vi "Format Geometric Patterns Results (SubVI).vi"(8 "error in":errorcluster, 11 "Matches":T1[](array[typedef]) {"Correlation Score" format="%.2f"; "Target Template Curve Score" format="%.2f"; "Template Target Curve Score" format="%.2f"; "Bounding Box"."y" format="%.2f"; "Bounding Box"."x" format="%.2f"; "Position"."y" format="%.2f"; "Position"."x" format="%.2f"; "Score" format="%.2f"; "Scale" format="%.2f"; "Angle" format="%.2f"; "Occlusion %" format="%.2f"}) -> (0 "error out":errorcluster, 3 "Text Results":string[][](table))   [LabVIEW 2016]
uses:
  <vilib>/vision/Pattern Matching.llb/IMAQ GM Match Report.ctl
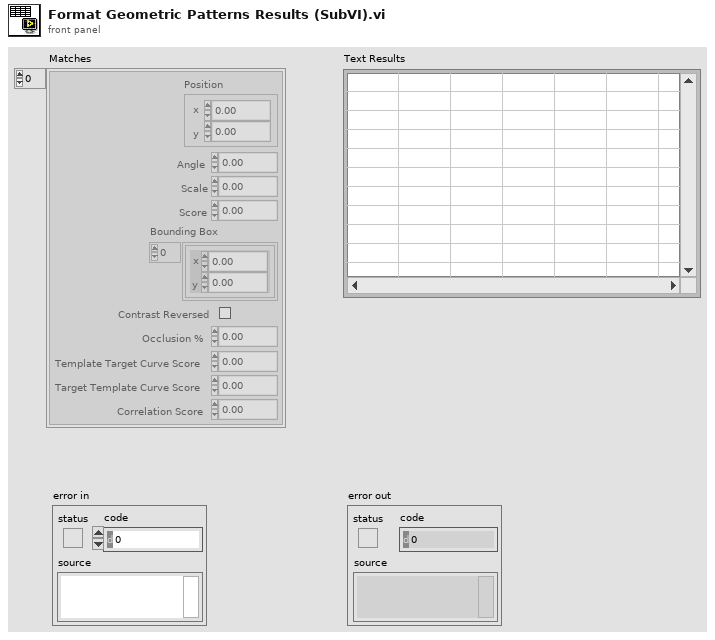
[diagram p1: front panel]
types:
  T1 = typedef "IMAQ GM Match Report.ctl" = cluster{"Position":cluster{"x":sgl, "y":sgl}, "Angle":sgl, "Scale":sgl, "Score":sgl, "Bounding Box":cluster{"x":sgl, "y":sgl}[], "Contrast Reversed":bool, "Occlusion %":sgl, "Template Target Curve Score":sgl, "Target Template Curve Score":sgl, "Correlation Score":sgl}
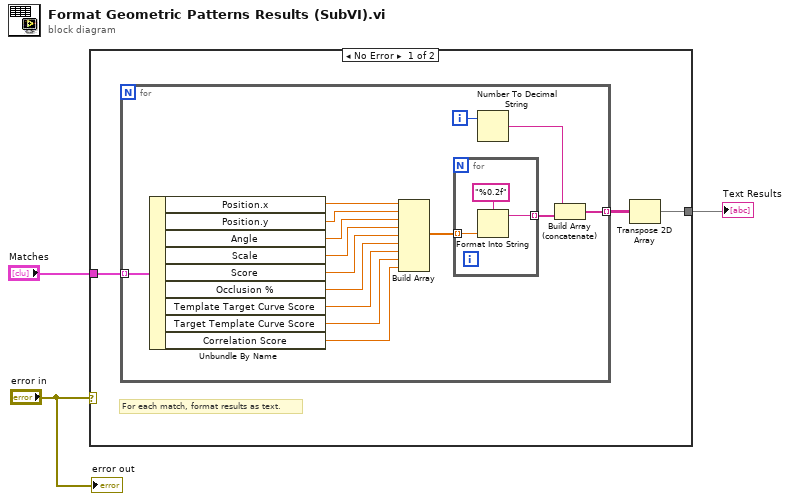
[diagram p0: block diagram]
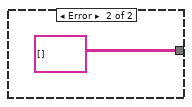
[diagram p2: hidden frame]
diagram:
  n1 = case shown="No Error" "error in" {
    tunnel: "Matches" -> [w6 _]
    tunnel: [w4 string[][] []] -> w2
    frame No Error {
      # "For each match, format results as text."
      n2 = for {
        tunnel: w6 -> [w21] mode=indexing
        tunnel: [w9] -> w5 mode=indexing
        i -> [w8]
        n3 = Unbundle By Name(w21) -> ("Position.x"=w20:sgl, "Position.y"=w19:sgl, "Angle"=w18:sgl, "Scale"=w17:sgl, "Score"=w16:sgl, "Occlusion %"=w15:sgl, "Template Target Curve Score"=w14:sgl, "Target Template Curve Score"=w13:sgl, "Correlation Score"=w12:sgl)
        n4 = Build Array(w20, w19, w18, w17, w16, w15, w14, w13, w12) -> (w11:sgl[])
        n5 = for {
          tunnel: w11 -> [w24] mode=indexing
          tunnel: [w22] -> w10 mode=indexing
          n6 = Format Into String(format string="%0.2f", w24) -> (resulting string=w22:string)  [unwired: 2 in, 1 out]
        }
        n7 = Number To Decimal String(number=w8) -> (decimal integer string=w7:string)  [unwired: 1 in]
        n8 = Build Array (concatenate)(w7, w10) -> (w9:string[])
      }
      n9 = Transpose 2D Array(2D array=w5) -> (transposed array=w4:string[][])
    }
    frame Error {
    }
  }
  "Text Results" <- w2
  "error out" <- "error in"
